vi "split_averaging_filter_nu.vi"(4 "Reset":bool, 8 "Parameters":T1={"Order"=0, "Time constant"=0.0, "Detrend mode"=enum."Robust linear", "TD amplitude limit"=inf, "FFT filter"=TRUE, "Notch channels"=[], "LF cutoff"=0, "FD amplitude limit"=0.0}, 9 "Noise":bool, 10 "Error mode":bool, 11 "Signal":dbl[](array[numeric])) -> (0 "Order variance":dbl[](array[numeric]), 1 "Order mean":dbl[](array[numeric]), 2 "Variance":dbl[](array[numeric]), 3 "Prediction":dbl[](array[numeric]))   [LabVIEW 2014]
uses:
  averaging_filter_params.ctl
  detrend_mode.ctl
  <vilib>/Analysis/2dsp.llb/Real FFT.vi
  <vilib>/Analysis/2dsp.llb/Inverse Real FFT.vi
  <vilib>/Analysis/NI_AALPro.lvlib
panel:
  in  "Update in Fourier domain.":bool
  # "Either full signal, or just filter tracking residue, depending on \"Error mode\""
  # "Prediction for next data block, the same size as our input this time."
  # "If true, previous \"Prediction\" has already been subtracted from \"Signal\".  If false, no time domain limiting is done.  (see note on block diagram about dual use for hum and distortion )"
  # "\"Order ...\" outputs are time domain models, with length \"Order\".   These are synchronous with the repeat period."
  # "If true, our adaptation should be suppressed on this \"Signal\" block."
  # "Reset clears state to zeroes.  Filter must then settle to the steady-state output (multiple time constants)."
  # "Mean and variance of a repeating signal with known repeat period (order).  Input may be any length; mean and variance outputs are the same size as input.  This is like the averaging function on an oscilliscope.  As long as the time constant is much longer than the filter order, only signals that are synchronous with the order pass through into the mean.   In the frequency domain, we pass the order and harmonics of it.\n\nVariance is the filtered mean-squared difference between the input and the mean. This represents the expected variation at each position in the repeat period."
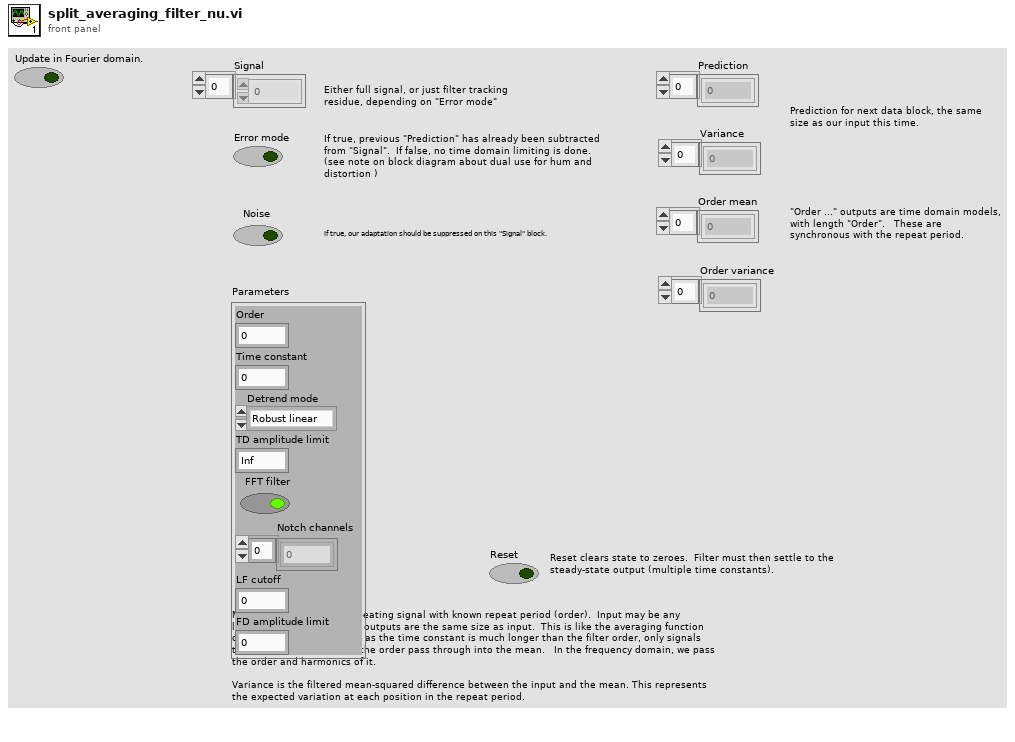
[diagram p1: front panel]
types:
  T1 = typedef "averaging_filter_params.ctl" = cluster{"Order":i32, "Time constant":dbl, "Detrend mode":T2, "TD amplitude limit":dbl, "FFT filter":bool, "Notch channels":i32[], "LF cutoff":i32, "FD amplitude limit":dbl}
  T2 = typedef "detrend_mode.ctl" = enum16{"Zero mean", "Linear", "Robust linear"}
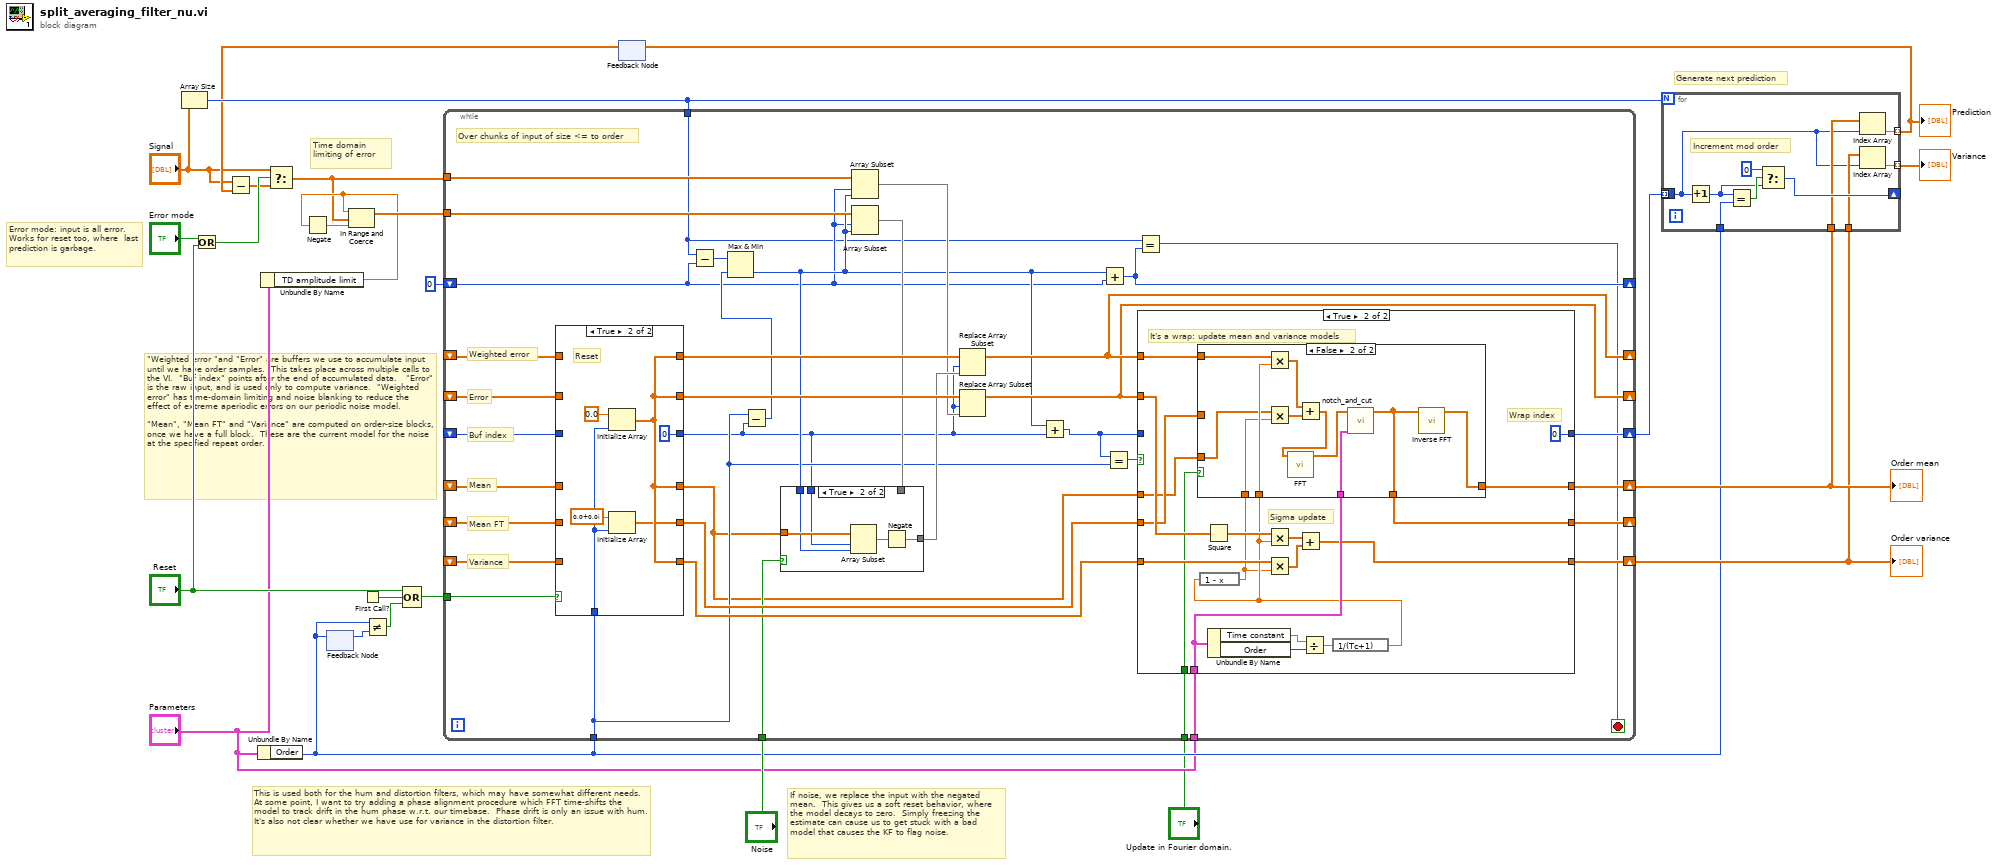
[diagram p0: block diagram]
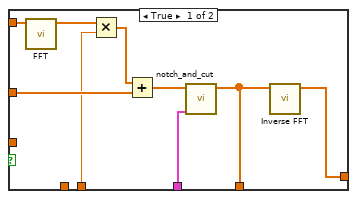
[diagram p5: hidden frame]
diagram:
  # "Error mode: input is all error.  Works for reset too, where  last prediction is garbage."
  # "Generate next prediction"
  # "If noise, we replace the input with the negated mean.  This gives us a soft reset behavior, where the model decays to zero.  Simply freezing the estimate can cause us to get stuck with a bad model that causes the KF to flag noise."
  # "\"Weighted error \"and \"Error\" are buffers we use to accumulate input until we have order samples.  This takes place across multiple calls to the VI.  \"Buf index\" points after the end of accumulated data.   \"Error\" is the raw input, and is used only to compute variance.  \"Weighted error\" has time-domain limiting and noise blanking to reduce the effect of extreme aperiodic errors on our periodic noise model. \n\n\"Mean\", \"Mean FT\" and \"Variance\" are computed on order-size blocks, once we have a full block.  These are the current model for the noise at the specified repeat order."
  # "Time domain limiting of error"
  # "This is used both for the hum and distortion filters, which may have somewhat different needs.  At some point, I want to try adding a phase alignment procedure which FFT time-shifts the model to track drift in the hum phase w.r.t. our timebase.  Phase drift is only an issue with hum.  It's also not clear whether we have use for variance in the distortion filter."
  n1 = Array Size(array="Signal") -> (size(s)=w14:i32)
  n2 = Or(x="Error mode", y="Reset") -> (x .or. y?=w6:bool)
  n3 = Unbundle By Name("Parameters") -> ("Order"=w19:i32)
  n4 = Unbundle By Name("Parameters") -> ("TD amplitude limit"=w7:dbl)
  n5 = Negate(x=w7) -> (-x=w8:dbl)
  n6 = feedback-in #1(w19) -> ()
  n7 = feedback #1() -> (w20:i32)  [unwired: 1 in]
  n8 = First Call?() -> (First Call?: T/F=w24:bool)
  n9 = Not Equal?(x=w19, y=w20) -> (x != y?=w18:bool)
  n10 = Compound Arithmetic op=OR("Reset", w24, w18) -> (w17:bool)
  n11 = feedback #2() -> (w5:dbl[])  [unwired: 1 in]
  n12 = Subtract(x="Signal", y=w5) -> (x-y=w4:dbl[])
  n13 = Select(t="Signal", s=w6, f=w4) -> (s? t:f=w2:dbl[])
  n14 = In Range and Coerce(upper limit=w7, x=w2, lower limit=w8) -> (coerced(x)=w10:dbl[])  [unwired: 1 out]
  n15 = while {
    shift-right: [w62] -> w16
    shift-left: _ -> [w51]
    tunnel: w19 -> [w30]
    shift-right: [w59] -> _
    shift-left: _ -> [w56]
    shift-right: [w60] -> w23
    shift-left: _ -> [w55]
    shift-right: [w37] -> _
    shift-left: _ -> [w52]
    shift-right: [w38] -> _
    shift-left: _ -> [w53]
    shift-right: [w58] -> w22
    shift-left: _ -> [w57]
    tunnel: "Parameters" -> [w61]
    tunnel: "Noise" -> [w42]
    tunnel: w17 -> [w54]
    tunnel: w10 -> [w47]
    shift-right: [w32] -> _
    shift-left: 0 ("Order") -> [w34]
    tunnel: w14 -> [w33]
    tunnel: w2 -> [w43]
    tunnel: "Update in Fourier domain." -> [w26]
    stop <- w31 stop-if-true
    # "Over chunks of input of size <= to order"
    # "Buf index"
    # "Mean FT"
    # "Error"
    # "Weighted error"
    # "Mean"
    # "Variance"
    n16 = case shown="True" w54 {
      tunnel: w30 -> [_ w76]
      tunnel: w56 -> [w74 _]
      tunnel: [w74 w75] -> w49
      tunnel: [w73 w77] -> w29
      tunnel: w55 -> [w73 _]
      tunnel: [w69 0 ("Order")] -> w28
      tunnel: [w70 w77] -> w46
      tunnel: [w71 w77] -> w45
      tunnel: [w72 w77] -> w50
      tunnel: w57 -> [w72 _]
      tunnel: w53 -> [w71 _]
      tunnel: w52 -> [w70 _]
      tunnel: w51 -> [w69 _]
      frame False {
        # "Not reset"
      }
      frame True {
        # "Reset"
        n17 = Initialize Array(0.0 ("Decay"), w76) -> (w77:dbl[])
        n18 = Initialize Array(cdb 0.0+0.0i ("Decay"), w76) -> (w75:cdb[])
      }
    }
    n19 = Subtract(x=w33, y=w34) -> (x-y=w48:i32)
    n20 = Subtract(x=w30, y=w28) -> (x-y=w44:i32)
    n21 = Max & Min(x=w48, y=w44) -> (min(x,y)=w35:i32)  [unwired: 1 out]
    n22 = Array Subset(array=w43, index=w34, length=w35) -> (w39:dbl[])
    n23 = Array Subset(array=w47, index=w34, length=w35) -> (w41:dbl[])
    n24 = case shown="True" w42 {
      tunnel: w41 -> [w63 _]
      tunnel: [w63 w64] -> w40
      tunnel: w29 -> [_ w68]
      tunnel: w28 -> [_ w67]
      tunnel: w35 -> [_ w66]
      frame False {
      }
      frame True {
        n25 = Array Subset(array=w68, index=w67, length=w66) -> (w65:dbl[])
        n26 = Negate(x=w65) -> (-x=w64:dbl[])
      }
    }
    n27 = Replace Array Subset(array=w45, new element=w40, index=w28) -> (w38:dbl[])
    n28 = Replace Array Subset(array=w46, new element=w39, index=w28) -> (w37:dbl[])
    n29 = Add(x=w35, y=w28) -> (x+y=w36:i32)
    n30 = Add(x=w35, y=w34) -> (x+y=w32:i32)
    n31 = Equal?(x=w36, y=w30) -> (x = y?=w27:bool)
    n32 = Equal?(x=w33, y=w32) -> (x = y?=w31:bool)
    n33 = case shown="True" w27 {
      tunnel: [w81 0] -> w62
      tunnel: w36 -> [w81 _]
      tunnel: w37 -> [_ w100]
      tunnel: w38 -> [_ w89]
      tunnel: w49 -> [w83 w99]
      tunnel: w61 -> [_ w93]
      tunnel: [w82 w98] -> w60
      tunnel: [w83 w97] -> w59
      tunnel: w50 -> [w84 w91]
      tunnel: [w84 w90] -> w58
      tunnel: w29 -> [w82 w85]
      tunnel: w26 -> [_ w87]
      frame False {
        # "Not a wrap"
      }
      frame True {
        # "Sigma update"
        # "Wrap index"
        # "It's a wrap: update mean and variance models"
        n34 = Square(x=w100) -> (x^2=w92:dbl[])
        n35 = Unbundle By Name(w93) -> ("Time constant"=w95:dbl, "Order"=w96:i32)
        n36 = Divide(x=w95, y=w96) -> (x/y=w94:dbl)
        n37 = expression code="1/(Tc+1)"(w94) -> (w88:dbl)
        n38 = expression code="1 - x"(w88) -> (w86:dbl)
        n39 = case shown="False" w87 {
          tunnel: w99 -> [w112 _]
          tunnel: [w111 w123] -> w98
          tunnel: [w110 w122] -> w97
          tunnel: w93 -> [w109 w121]
          tunnel: w89 -> [w108 w118]
          tunnel: w88 -> [w104 w119]
          tunnel: w86 -> [_ w117]
          tunnel: w85 -> [_ w115]
          frame True {
            n40 = call-poly <vilib>:"FFT.vi"("X"=w108) -> ("FFT {X}"=w107:cdb[])  [unwired: 9 in, 1 out]
            n41 = Multiply(x=w107, y=w104) -> (x*y=w106:cdb[])
            n42 = Add(x=w106, y=w112) -> (x+y=w105:cdb[])
            n43 = call "notch_and_cut.vi"("Parameters"=w109, "In"=w105) -> ("Out"=w110:cdb[])  [unwired: 9 in]
            n44 = call-poly <vilib>:"Inverse FFT.vi"("FFT {X}"=w110) -> ("X"=w111:dbl[])  [unwired: 9 in, 1 out]
          }
          frame False {
            n45 = Multiply(x=w118, y=w119) -> (x*y=w120:dbl[])
            n46 = Multiply(x=w115, y=w117) -> (x*y=w116:dbl[])
            n47 = Add(x=w120, y=w116) -> (x+y=w114:dbl[])
            n48 = call-poly <vilib>:"FFT.vi"("X"=w114) -> ("FFT {X}"=w113:cdb[])  [unwired: 9 in, 1 out]
            n49 = call "notch_and_cut.vi"("Parameters"=w121, "In"=w113) -> ("Out"=w122:cdb[])  [unwired: 9 in]
            n50 = call-poly <vilib>:"Inverse FFT.vi"("FFT {X}"=w122) -> ("X"=w123:dbl[])  [unwired: 9 in, 1 out]
          }
        }
        n51 = Multiply(x=w92, y=w88) -> (x*y=w101:dbl[])
        n52 = Multiply(x=w91, y=w86) -> (x*y=w102:dbl[])
        n53 = Add(x=w101, y=w102) -> (x+y=w90:dbl[])
      }
    }
  }
  "Order mean" <- w23
  "Order variance" <- w22
  n54 = for {
    N: w14 -> [_]
    shift-right: [w129] -> _
    shift-left: w16 -> [w124]
    tunnel: w19 -> [w132]
    tunnel: [w127] -> w13 mode=indexing
    tunnel: [w128] -> w25 mode=indexing
    tunnel: w22 -> [w126]
    tunnel: w23 -> [w125]
    tunnel: [w124] -> _ mode=indexing
    # "Increment mod order"
    n55 = Increment(x=w124) -> (x+1=w131:i32)
    n56 = Equal?(x=w131, y=w132) -> (x = y?=w133:bool)
    n57 = Select(t=0, s=w133, f=w131) -> (s? t:f=w129:i32)
    n58 = Index Array(array=w125, index=w124) -> (element=w127:dbl)
    n59 = Index Array(array=w126, index=w124) -> (element=w128:dbl)
  }
  "Prediction" <- w13
  "Variance" <- w25
  n60 = feedback-in #2(w13) -> ()
